vi "e.gate ASCII Error Handler.vi"(8 "error in (no error)":errorcluster, 11 "String":string) -> (0 "error out":errorcluster)   [LabVIEW 2016]
doc: "<B>AMC - Analytik & Messtechnik GmbH Chemnitz</B>\n\nLabVIEW Drivers for e.gate / e.pac series from Gantner Instruments\n\nThis VI throws a LabVIEW error if the device response is NACK."
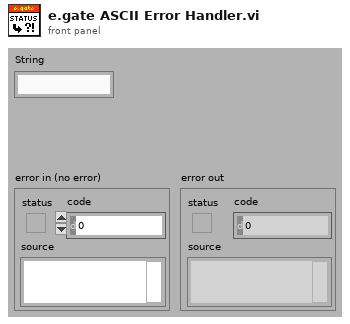
[diagram p1: front panel]
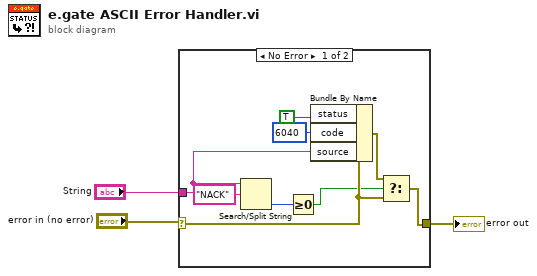
[diagram p0: block diagram]
diagram:
  n1 = case shown="No Error" "error in (no error)" {
    selector: "error in (no error)" -> [w11 w13]
    tunnel: "String" -> [w7 _]
    tunnel: [w12 w13] -> w1
    frame No Error {
      n2 = Search/Split String(string=w7, search string/char (-)="NACK") -> (offset of match=w5:i32)  [unwired: 3 out]
      n3 = Greater Or Equal To 0?(x=w5) -> (x >= 0?=w4:bool)
      n4 = Bundle By Name(cluster=w11, "status"=TRUE, "code"=6040, "source"=w7) -> (w8:errorcluster)
      n5 = Select(t=w8, s=w4, f=w11) -> (s? t:f=w12:errorcluster)
    }
    frame Error {
    }
  }
  "error out" <- w1
